vi "Set Table Record.vi"(1 "Data In":T1) -> (0 "Record Out":string[](array[string]))   [LabVIEW 2018]
uses:
  Ctls/DisplayIndicator.ctl
  Ctls/MotroConfigData.ctl
  Ctls/MotorConfig.ctl
  Ctls/MagType.ctl
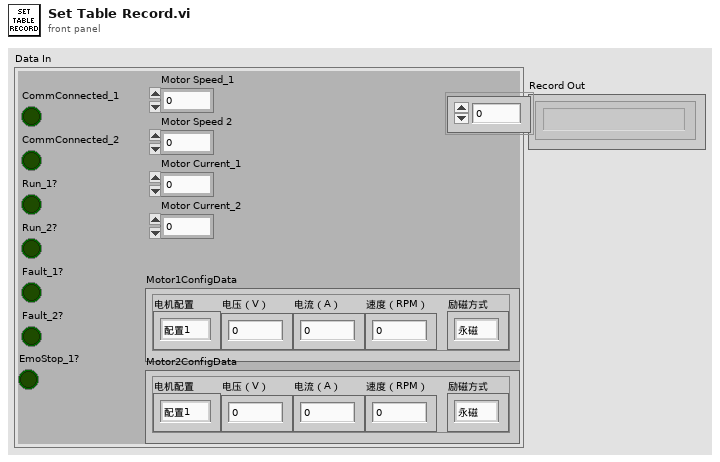
[diagram p1: front panel]
types:
  T1 = typedef "DisplayIndicator.ctl" = cluster{"CommConnected_1":bool, "Run_1?":bool, "Fault_1?":bool, "CommConnected_2":bool, "Run_2?":bool, "Fault_2?":bool, "Motor Speed 2":sgl, "Motor Speed_1":sgl, "Motor Current_1":sgl, "Motor Current_2":sgl, "Motor1ConfigData":T2, "Motor2ConfigData":T2, "EmoStop_1?":bool}
  T2 = typedef "MotroConfigData.ctl" = cluster{"电机配置":T3, "电压（V）":dbl, "电流（A）":dbl, "速度（RPM）":dbl, "励磁方式":T4}
  T3 = typedef "MotorConfig.ctl" = enum16{"配置1", "配置2", "配置3", "配置4"}
  T4 = typedef "MagType.ctl" = enum16{"永磁", "励磁"}
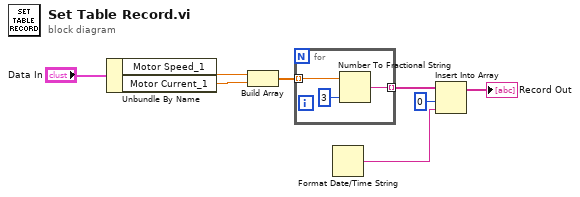
[diagram p0: block diagram]
diagram:
  n1 = Unbundle By Name("Data In") -> ("Motor Speed_1"=w4:sgl, "Motor Current_1"=w5:sgl)
  n2 = Build Array(w4, w5) -> (w6:sgl[])
  n3 = for {
    tunnel: w6 -> [w10] mode=indexing
    tunnel: [w9] -> w7 mode=indexing
    n4 = Number To Fractional String(number=w10, precision (6)=i16 3) -> (F-format string=w9:string)  [unwired: 2 in]
  }
  n5 = Format Date/Time String() -> (date/time string=w1:string)  [unwired: 3 in]
  n6 = Insert Into Array(array=w7, index=0, new element=w1) -> (→"Record Out":string[])
